vi "db.vi"(10 "AuditorID":string) -> (2 "Eventos":string[][](array[string]))   [LabVIEW 2012]
uses:
  <vilib>/addons/database/Auxilliary.llb/DB Tools Cursor Type.ctl
  <vilib>/addons/database/Connection.llb/DB Tools Open Connec (Path).vi
  <vilib>/addons/database/Connection.llb/Conn Execute.vi
  <vilib>/addons/database/Recordset.llb/Rec Fetch Recordset Data (R).vi
  <vilib>/addons/database/Recordset.llb/Rec Destroy - Connection.vi
  <vilib>/addons/database/_DB Variant To Data/Database Variant To Data.xnode
  <vilib>/addons/database/NI_Database_API.lvlib
panel:
  out "string":string
  out "POC":string[](array[string])
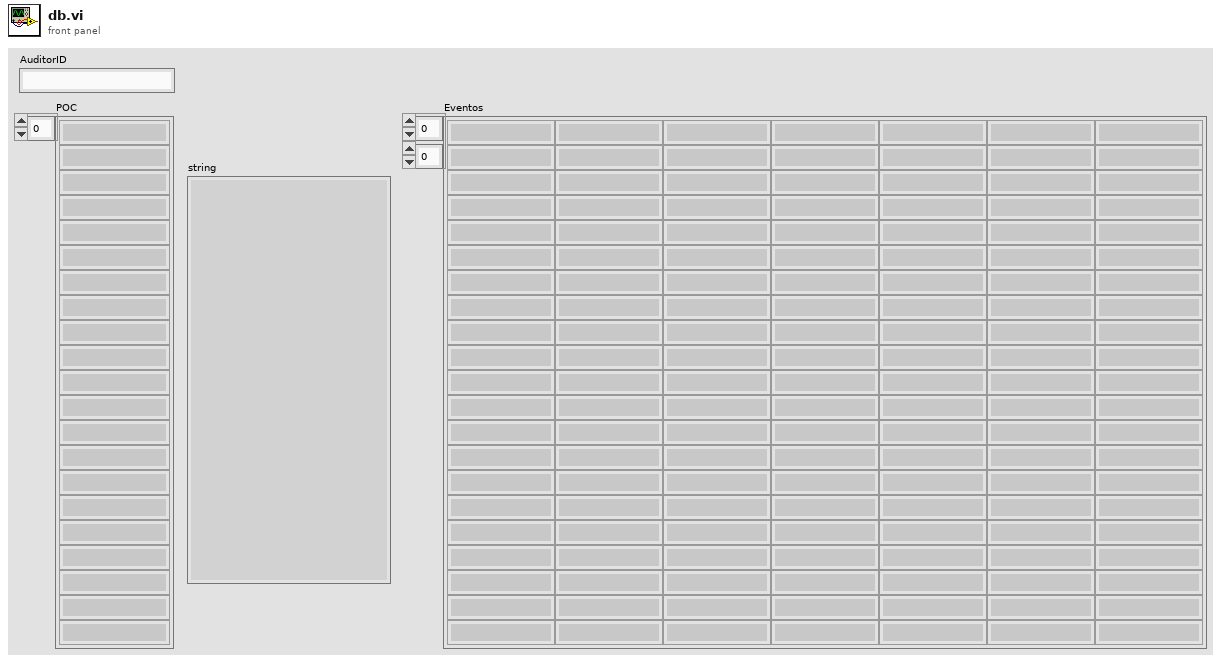
[diagram p1: front panel]
types:
  T1 = enum16{"POC", "Imei", "Evento", "Lat", "Lon", "F_H_eve", "F_H_rec", "AVL_N", "AVL_pass", "Propietario", "Razon_Social", "Direccion", "Propietario_N", "Ciudad", "Marca", "Ruta", "N_Ruta", "Auditor_ST", "Auditor_P", "Auditor_N"}
  T2 = enum16{"POC", "Imei", "Evento", "Lat", "Lon", "F_H_eve", "F_H_rec", "AVL_N", "AVL_pass", "Propietario", "Razon_Social", "Direccion", "Propietario_N", "Ciudad", "Marca", "Ruta", "N_Ruta", "Auditor", "Auditor_N"}
  T3 = typedef "NI_Database_API.lvlib/DB Tools Cursor Type.ctl" = enum16{"forward-only", "keyset", "dynamic", "static"}
  T4 = typedef "NI_Database_API.lvlib/Conn ObjectReference.ctl" = refnum<k1>
  T5 = typedef "NI_Database_API.lvlib/Rec ObjectReference.ctl" = refnum<k1>
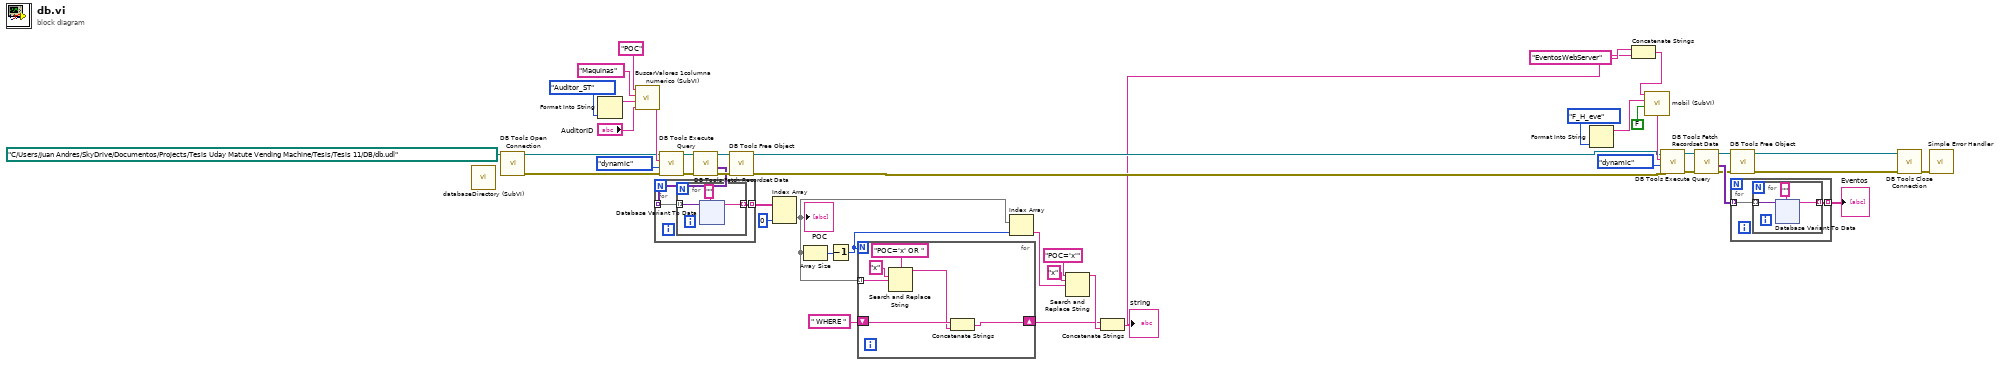
[diagram p0: block diagram]
diagram:
  n1 = call "databaseDirectory (SubVI).vi"() -> ()  [unwired: 1 in, 1 out]
  n2 = call-poly <vilib>:"DB Tools Open Connection.vi"("connection information"=path "C:/Users/Juan Andres/SkyDrive/Documentos/Projects/Tesis Uday Matute Vending Machine/Tesis/Tesis 11/DB/db.udl") -> ("error out"=w15:errorcluster, "connection reference"=w16:T4)  [unwired: 7 in]
  n3 = Format Into String(T1."Auditor_ST") -> (resulting string=w35:string)  [unwired: 3 in, 1 out]
  n4 = call "BuscarValores 1columna numerico (SubVI).vi"("Columna?"="POC", "Tabla"="Maquinas", "Columna"=w35, "="="AuditorID") -> ("String"=w37:string)  [unwired: 6 in]
  n5 = call-poly <vilib>:"DB Tools Execute Query.vi"("error in (no error)"=w15, "cursor type"=DB_Tools_Cursor_Type."dynamic", "SQL query"=w37, "connection reference"=w16) -> ("error out"=w41:errorcluster, "recordset reference"=w42:T5)  [unwired: 4 in]
  n6 = call-poly <vilib>:"DB Tools Fetch Recordset Data.vi"("error in (no error)"=w41, "recordset reference"=w42) -> ("error out"=w39:errorcluster, "recordset data"=w33:variant[][], "recordset reference out"=w40:T5)  [unwired: 3 in]
  n7 = for {
    tunnel: w33 -> [w47] mode=indexing
    tunnel: [w46] -> w32 mode=indexing
    n8 = for {
      tunnel: w47 -> [w49] mode=indexing
      tunnel: [w48] -> w46 mode=indexing
      n9 = xnode "Database Variant To Data"("database variant"=w49, "type"="") -> ("data"=w48:string)  [unwired: 1 in, 1 out]
    }
  }
  n10 = call-poly <vilib>:"DB Tools Free Object.vi"("error in (no error)"=w39, "recordset reference"=w40) -> ("error out"=w13:errorcluster, "connection reference"=w14:T4)  [unwired: 8 in]
  n11 = Index Array(array=w32, index (col)=0 ("disabled index (col)")) -> (element=w8:string[])  [unwired: 1 in]
  "POC" <- w8
  n12 = Array Size(array=w8) -> (size(s)=w9:i32)
  n13 = Decrement(x=w9) -> (x-1=w2:i32)
  n14 = for {
    N: w2 -> [_]
    tunnel: w8 -> [w86] mode=indexing
    shift-right: [w83] -> w3
    shift-left: " WHERE " ("string") -> [w85]
    n15 = Search and Replace String(input string="POC='x' OR " ("string"), search string="x", replace string=w86) -> (result string=w84:string)  [unwired: 5 in, 3 out]
    n16 = Concatenate Strings(w85, w84) -> (w83:string)
  }
  n17 = Index Array(array=w8, index=w2) -> (element=w5:string)
  n18 = Search and Replace String(input string="POC='x'" ("string"), search string="x", replace string=w5) -> (result string=w4:string)  [unwired: 5 in, 3 out]
  n19 = Concatenate Strings(w3, w4) -> (w1:string)
  "string" <- w1
  n20 = Format Into String(T2."F_H_eve") -> (resulting string=w21:string)  [unwired: 3 in, 1 out]
  n21 = Concatenate Strings("EventosWebServer" ("Tabla"), w1) -> (w11:string)
  n22 = call "mobil (SubVI).vi"("Orden"=FALSE, "Columna"=w21, "Tabla"=w11) -> ("String"=w23:string)  [unwired: 8 in]
  n23 = call-poly <vilib>:"DB Tools Execute Query.vi"("error in (no error)"=w13, "cursor type"=DB_Tools_Cursor_Type."dynamic", "SQL query"=w23, "connection reference"=w14) -> ("error out"=w25:errorcluster, "recordset reference"=w24:T5)  [unwired: 4 in]
  n24 = call-poly <vilib>:"DB Tools Fetch Recordset Data.vi"("error in (no error)"=w25, "recordset reference"=w24) -> ("error out"=w27:errorcluster, "recordset data"=w30:variant[][], "recordset reference out"=w26:T5)  [unwired: 3 in]
  n25 = call-poly <vilib>:"DB Tools Free Object.vi"("error in (no error)"=w27, "recordset reference"=w26) -> ("error out"=w43:errorcluster, "connection reference"=w44:T4)  [unwired: 8 in]
  n26 = for {
    tunnel: w30 -> [w90] mode=indexing
    tunnel: [w89] -> w17 mode=indexing
    n27 = for {
      tunnel: w90 -> [w92] mode=indexing
      tunnel: [w91] -> w89 mode=indexing
      n28 = xnode "Database Variant To Data"("database variant"=w92, "type"="") -> ("data"=w91:string)  [unwired: 1 in, 1 out]
    }
  }
  "Eventos" <- w17
  n29 = call <vilib>:"DB Tools Close Connection.vi"("error in (no error)"=w43, "connection reference"=w44) -> ("error out"=w45:errorcluster)  [unwired: 5 in]
  n30 = call <vilib>:"Simple Error Handler.vi"("error in (no error)"=w45) -> ()  [unwired: 4 in, 5 out]
